vi "TDMS File Viewer.vi"() -> ()   [LabVIEW 2023, in "GettingStarted_Common_148X_Host.lvlib"]
uses:
  GettingStarted_Common_148X_Host.lvlib
  Types/Packet Table.ctl
  <vilib>/Utility/miscctls.llb/LVRowAndColumnUnsignedTypeDef.ctl
panel:
  in  "Update TDMS File Packet Offset Data":bool
  in  "Packets to Display":i64=-1
  in  "Packet Display Start Index":u64
  out "Packets":T1
  out "Number of Packets in File":i64
  in  "serial input channel":string="SI0"
  in  "TDMS File Directory":path
  out "Error Out":errorcluster
  # "Overview: View the packet contents of a TDMS file containing acquired CSI-2 data and timestamps.  \nRequirements: FlexRIO\nInstructions: \n 1. Enter the name of the serial channel used to acquire the data.  This is used to construct the file names used with the CSI-2 Getting Started Examples.\n 2. Select the directory containing the TDMS file to read.\n 3. Set Packet Display Start Index to select the offset of the first packet to display.\n 4. Select the number of packets to display.  A negative value or a value larger than the remaining data in the file will read to to the end of file.\n 5. If the file does not contain packet offset data, enable the Update TDMS File Packet Offset Data control to add offsets. Keep disabled if the TDMS file already contains packet offset data. Offsets can reduce load time, particularly when reading a subset of the packet data.\n 6. Run the VI."
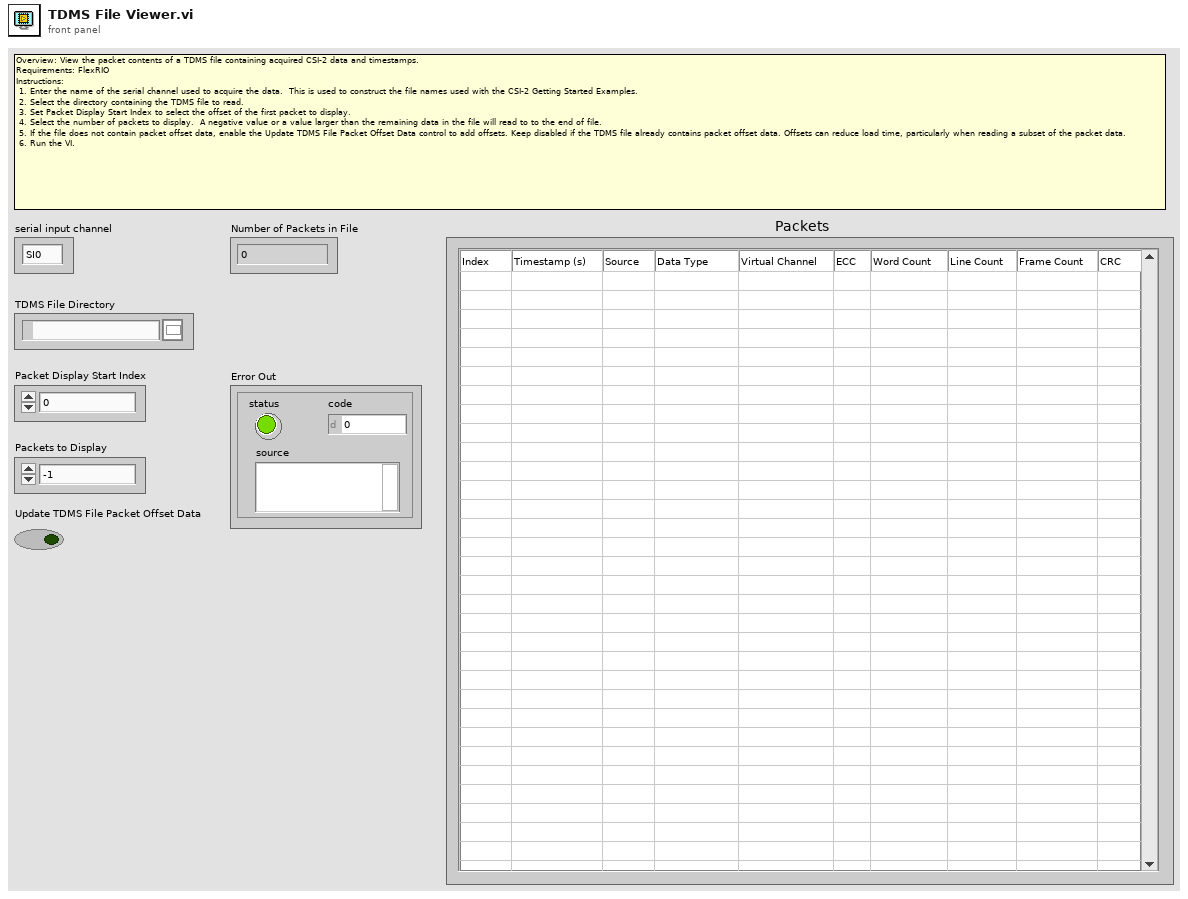
[diagram p1: front panel]
types:
  T1 = typedef "GettingStarted_Common_148X_Host.lvlib/Packet Table.ctl" = string[][]
  T2 = typedef "LVRowAndColumnUnsignedTypeDef.ctl" = cluster{"Row":u32, "Column":u32}
  T3 = typedef "NI CSI-2 API Host v2.lvlib/Host Tagged LLP Packet.ctl" = cluster{"tag":T4, "llp packet":T8}
  T4 = typedef "NI CSI-2 API Host v2.lvlib/Host LLP Packet Tag.ctl" = cluster{"timestamp":T5, "size":T7}
  T5 = typedef "NI CSI-2 API Host v2.lvlib/Host LLP Packet Timestamp.ctl" = cluster{"valid":bool, "count":u64, "id":T6, "metadata":u8}
  T6 = typedef "NI CSI-2 API FPGA v2.lvlib/Timestamp ID.ctl" = enum8{"SI0 LLP", "SI1 LLP", "SI2 LLP", "SI3 LLP", "SI4 LLP", "SI5 LLP", "SI6 LLP", "SI7 LLP", "SO0 LLP", "SO1 LLP", "SO2 LLP", "SO3 LLP", "SO4 LLP", "SO5 LLP", "SO6 LLP", "SO7 LLP", "Ser0 GPIO Bank", "Ser1 GPIO Bank", "Ser2 GPIO Bank", "Ser3 GPIO Bank", "Ser4 GPIO Bank", "Ser5 GPIO Bank", "Ser6 GPIO Bank", "Ser7 GPIO Bank", "Des0 GPIO Bank", "Des1 GPIO Bank", "Des2 GPIO Bank", "Des3 GPIO Bank", "Des4 GPIO Bank", "Des5 GPIO Bank", "Des6 GPIO Bank", "Des7 GPIO Bank", "User0", "User1", "User2", "User3", "User4", "User5", "User6", "User7", "User8", "User9", "User10", "User11", "User12", "User13", "User14", "User15", "User16", "User17", "User18", "User19", "User20", "User21", "User22", "User23", "User24", "User25", "User26", "User27", "User28", "User29", "User30", "User31"}
  T7 = typedef "NI CSI-2 API Host v2.lvlib/Host LLP Packet Size.ctl" = cluster{"bytes":u32, "valid":bool}
  T8 = typedef "NI CSI-2 API Host v2.lvlib/Host LLP Packet.ctl" = cluster{"header":T9, "payload":u8[], "footer":T10}
  T9 = typedef "NI CSI-2 API FPGA v2.lvlib/LLP Packet Header.ctl" = cluster{"word count":u16, "ecc":fxp<+,6,6>, "vcx":fxp<+,2,2>, "data type":fxp<+,6,6>, "vc":fxp<+,2,2>}
  T10 = typedef "NI CSI-2 API FPGA v2.lvlib/LLP Packet Footer.ctl" = cluster{"crc":u16}
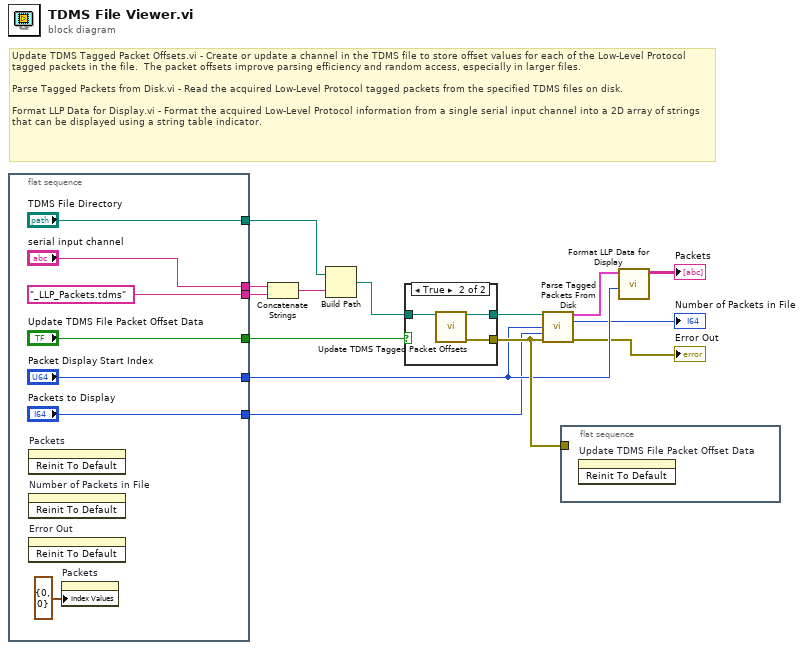
[diagram p0: block diagram]
diagram:
  # "Update TDMS Tagged Packet Offsets.vi - Create or update a channel in the TDMS file to store offset values for each of the Low-Level Protocol tagged packets in the file.  The packet offsets improve parsing efficiency and random access, especially in larger files.\n\nParse Tagged Packets from Disk.vi - Read the acquired Low-Level Protocol tagged packets from the specified TDMS files on disk. \n\nFormat LLP Data for Display.vi - Format the acquired Low-Level Protocol information from a single serial input channel into a 2D array of strings that can be displayed using a string table indicator."
  n1 = flat-sequence {
    tunnel: ["_LLP_Packets.tdms"] -> w11
    tunnel: ["TDMS File Directory"] -> w10
    tunnel: ["serial input channel"] -> w9
    tunnel: ["Packet Display Start Index"] -> w8
    tunnel: ["Packets to Display"] -> w7
    tunnel: ["Update TDMS File Packet Offset Data"] -> w1
    frame #0 {
      n2 = invoke on="Packets" class="Tbl (strict)" method="Reinit To Default"() -> ()  [unwired: 3 in, 3 out]
      n3 = invoke on="Number of Packets in File" class="DigNum (strict)" method="Reinit To Default"() -> ()  [unwired: 3 in, 3 out]
      n4 = invoke on="Error Out" class="Clust (strict)" method="Reinit To Default"() -> ()  [unwired: 3 in, 3 out]
      n5 = property on="Packets" class="Tbl (strict)"("Index Values"=T2 {"Row"=0, "Column"=0}) -> ()  [unwired: 2 in, 2 out]
    }
  }
  n6 = Concatenate Strings(w9, w11) -> (w12:string)
  n7 = Build Path(base path=w10, name or relative path=w12) -> (appended path=w3:path)
  n8 = case shown="True" w1 {
    tunnel: w3 -> [w22 w25]
    tunnel: [_ w24] -> w14
    tunnel: [w22 w23] -> w2
    frame False {
    }
    frame True {
      n9 = call "Update TDMS Tagged Packet Offsets.vi"("llp tagged packet file path"=w25) -> ("llp tagged packet file path out"=w23:path, "error out"=w24:errorcluster)  [unwired: 13 in]
    }
  }
  n10 = call "Parse Tagged Packets From Disk.vi"("llp tagged packet file path"=w2, "packet start index"=w8, "num packets to read"=w7, "error in"=w14) -> ("tagged packets"=w6:T3[], "total packets in file"=→"Number of Packets in File":i64, "error out"=→"Error Out":errorcluster)  [unwired: 8 in, 1 out]
  n11 = flat-sequence {
    tunnel: w14 -> [_]
    frame #0 {
      n12 = invoke on="Update TDMS File Packet Offset Data" class="Bool (strict)" method="Reinit To Default"() -> ()  [unwired: 3 in, 3 out]
    }
  }
  n13 = call "Format LLP Data for Display.vi"("packet index offset"=w8, "tagged packets"=w6) -> ("display data"=→"Packets":string[][])  [unwired: 9 in]
